vi "Curve fitting.vi"() -> ()   [LabVIEW 2016]
uses:
  <vilib>/Analysis/6fits.llb/Curve Fitting Criteria.ctl
  <vilib>/Analysis/NI_AALPro.lvlib
panel:
  in  "X3":dbl=0.3
  in  "Make it last element ?":bool
  in  "X1":dbl=-0.30000000000000004
  in  "Make it first element ?":bool
  out "Barrier array":dbl[](array[numeric])=[0.3892987340143991]
  in  "X2":dbl
  out "All X for plotting tangent curves":dbl[](array[numeric])=[-0.371549214007658, -8.080417881800293e-06, -0.30000808041805316, 0.29999191958211435, 0.37184895960201303]
  out "XY Graph":cluster{dbl[], dbl[]}[](graph)
  in  "X Array for plotting tangent curves":dbl[](array[numeric])=[0.0, -0.30000000000000004, 0.30000000000000004]
  out "Data section you choose":cluster{dbl[], "Best Polynomial Fit":dbl[]}[](graph)
  in  "Section selection":enum32{"Curve Array section", "Curve section"}(tab)
  in  "Sec of curve array ?":bool=TRUE
  in  "Starting":i32
  in  "length":i32=1
  out "Data array size(s)":i32=6
  in  "length":i32=5012
  in  "Starting":i32=2389
  out "size per curve":i32=4999
  in  "Section of curve ?":bool
  in  "Fitting type":T1(ring)
  in  "method (least square is default)":T2 items=["Least Square", "Least Absolute Residual", "Bisquare"]
  out "Fitting Coefficients":dbl[][](array[numeric])=[[6.3242027435342765e-12, 1.736578525198794e-09, -6.226360766319523e-10, 8.347622973355356e-09, 2.6562376943384554e-08, 1.896167754824949e-07]] format="%#_6p"
  in  "Original data curves":cluster{dbl[], dbl[]}[](graph)=[{array[4999 elements], array[4999 elements]}, {array[4999 elements], array[4999 elements]}, {array[4999 elements], array[4999 elements]}, {array[4999 elements], array[4999 elements]}, {array[4999 elements], array[4999 elements]}, {array[4999 elements], array[4999 elements]}]
  in  "polynomial order":i32=5
  out "Fitting curves":cluster{dbl[], "Best Polynomial Fit":dbl[]}[](graph)
  # "For polynomial fitting: Row is the fitting parameter for each curve (from 0th order to nth order).\nFor exponential fitting: Row is the fitting parameter for each curve (amp, damping, offset -- a,b,c for y=a*exp(bx)+c)."
  # "X difference between intersection of tangent curve at X1 & X2 and intersection of tangent curve at X2 & X3"
  # "Choose range of curve array"
  # "Choose range of each curve"
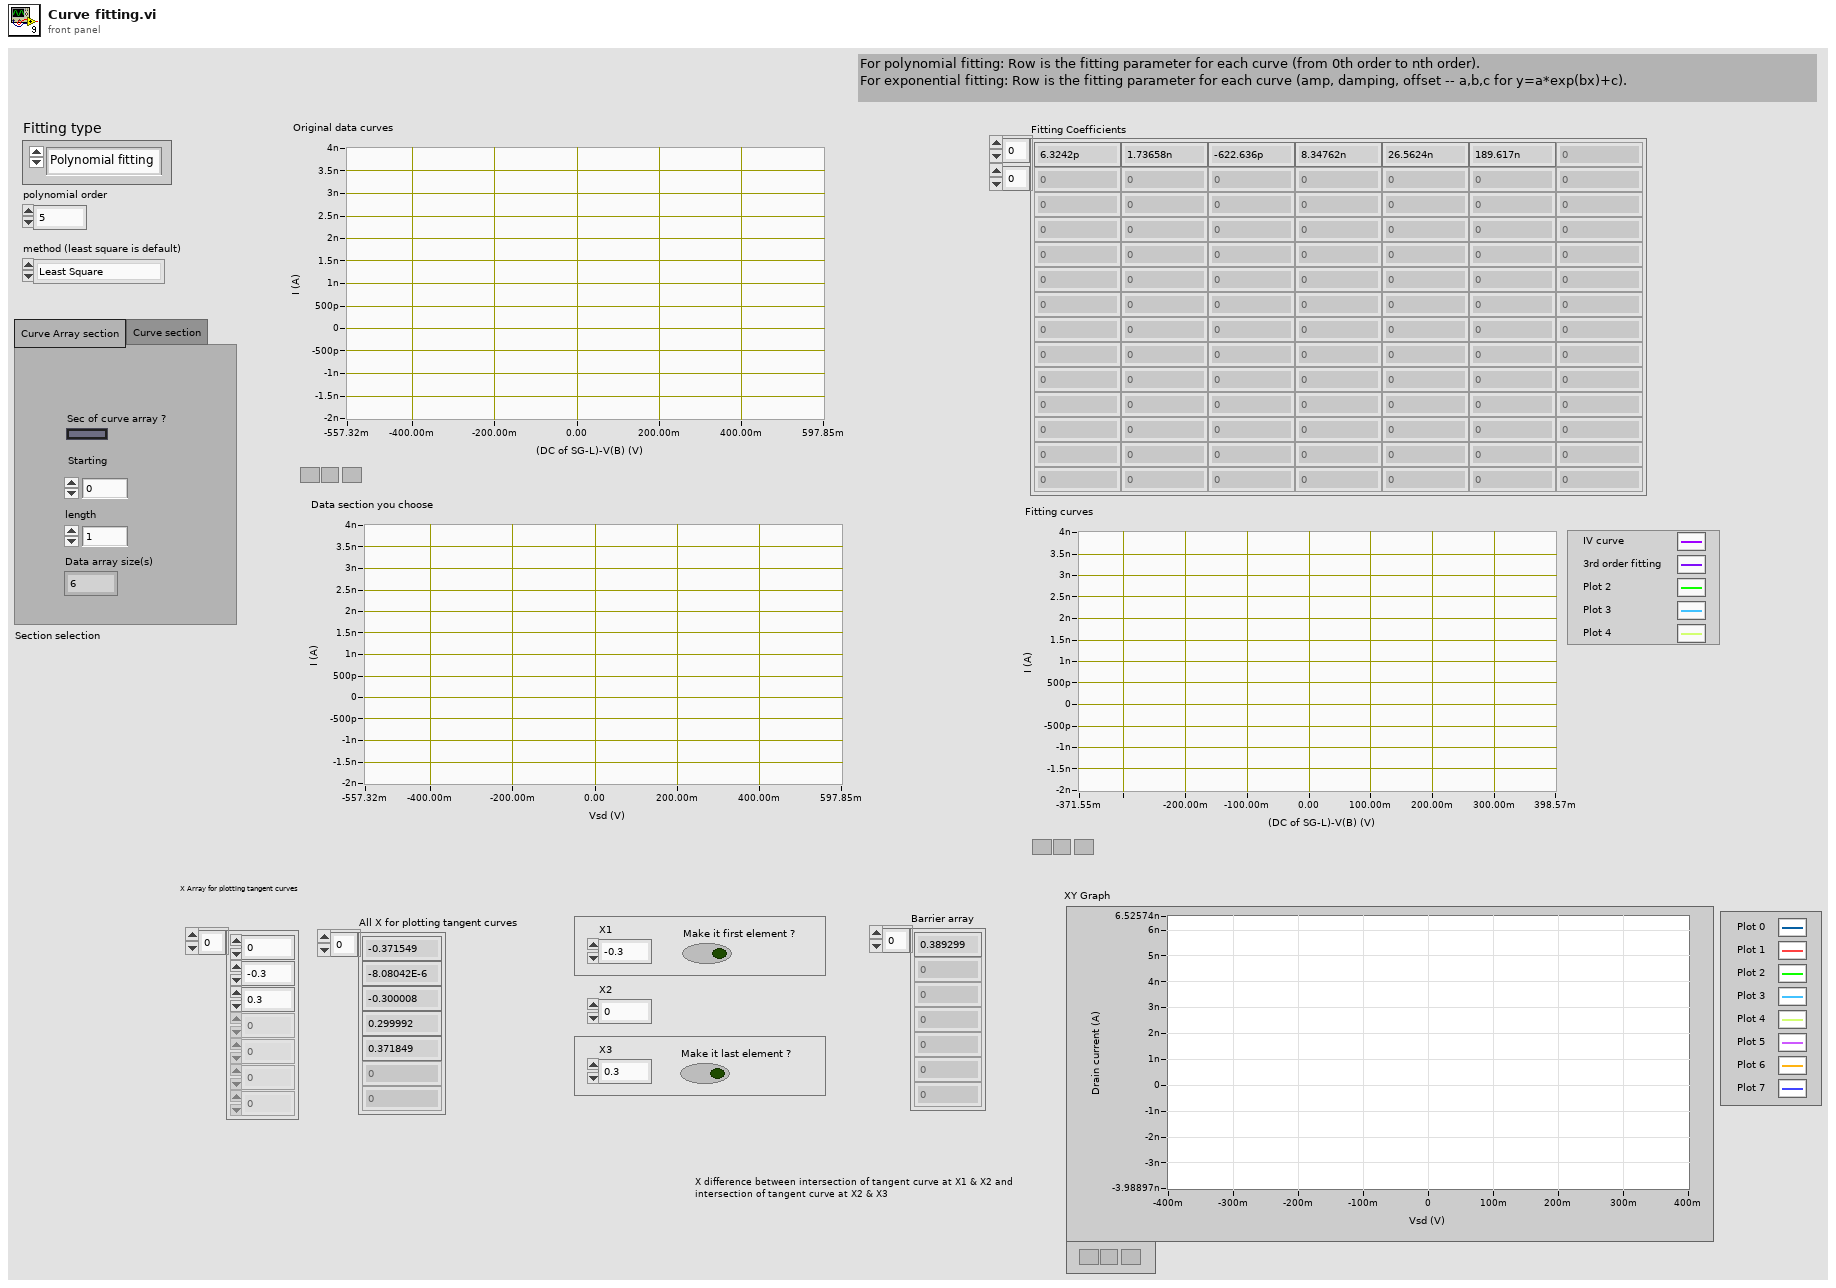
[diagram p1: front panel]
types:
  T1 = enum16{"Polynomial fitting", "Exponential fitting"}
  T2 = typedef "NI_AALPro.lvlib/Curve Fitting Criteria.ctl" = u16
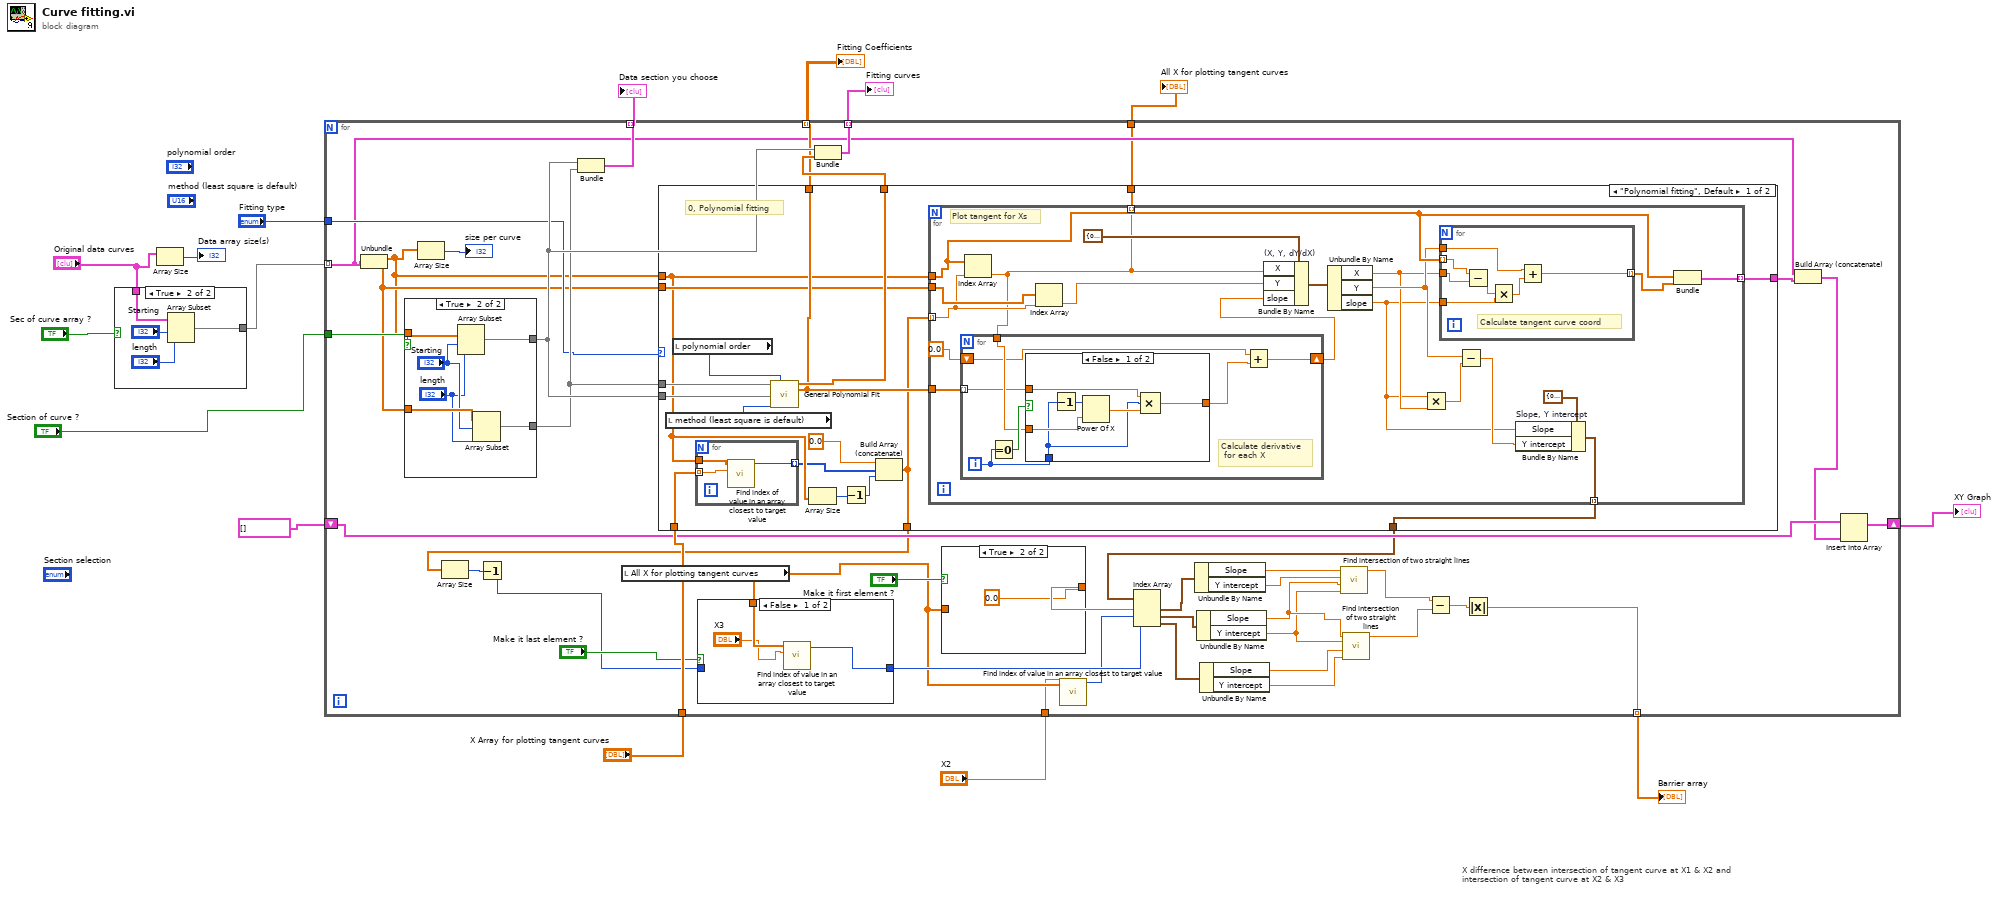
[diagram p0: block diagram]
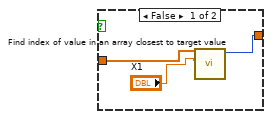
[diagram p4: hidden frame]
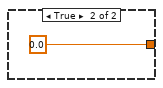
[diagram p5: hidden frame]
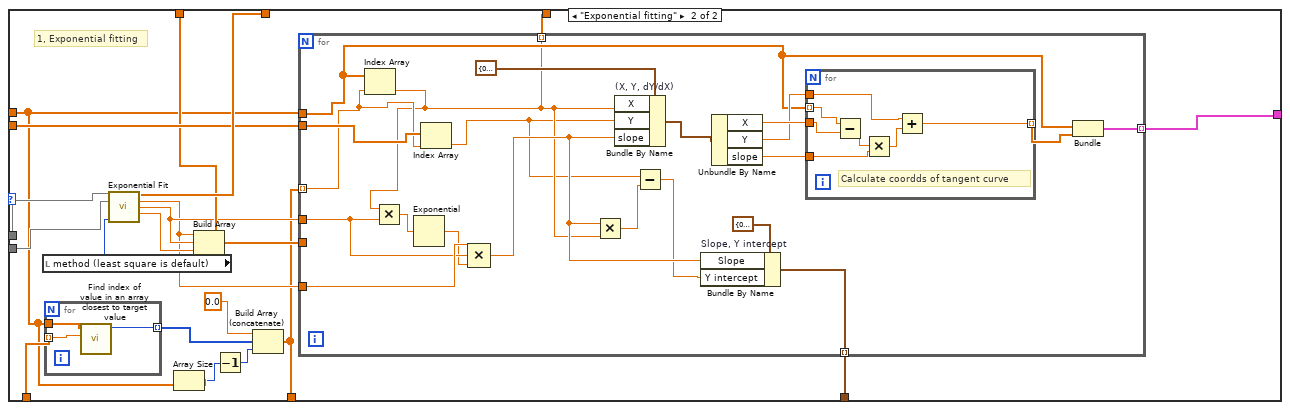
[diagram p6: hidden frame]
diagram:
  # "X difference between intersection of tangent curve at X1 & X2 and intersection of tangent curve at X2 & X3"
  n1 = case shown="True" "Sec of curve array ?" {
    tunnel: "Original data curves" -> [w16 w20]
    tunnel: [w16 w17] -> w10
    frame False {
    }
    frame True {
      n2 = Array Subset(array=w20, index="Starting", length="length") -> (w17:cluster{dbl[], dbl[]}[])
    }
  }
  n3 = Array Size(array="Original data curves") -> (size(s)=→"Data array size(s)":i32)
  n4 = for {
    tunnel: [w54] -> w14 mode=indexing
    tunnel: [w61] -> w15 mode=indexing
    tunnel: w10 -> [w50] mode=indexing
    tunnel: "Fitting type" -> [w53]
    tunnel: "Section of curve ?" -> [w59]
    tunnel: [w56] -> w7 mode=indexing
    tunnel: "X Array for plotting tangent curves" -> [w55]
    shift-right: [w46] -> w4
    shift-left: cluster{dbl[], dbl[]}[] [] ("appended array") -> [w48]
    tunnel: [w45] -> w3
    tunnel: "X2" -> [w23]
    tunnel: [w33] -> w1 mode=indexing
    n5 = Unbundle(w50) -> (w51:dbl[], w52:dbl[])
    n6 = case shown="True" w59 {
      tunnel: w51 -> [w182 w188]
      tunnel: [w182 w187] -> w58
      tunnel: w52 -> [w181 w186]
      tunnel: [w181 w183] -> w57
      frame False {
      }
      frame True {
        n7 = Array Subset(array=w188, index="Starting", length="length") -> (w187:dbl[])
        n8 = Array Subset(array=w186, index="Starting", length="length") -> (w183:dbl[])
      }
    }
    n9 = Array Size(array=w51) -> (size(s)=→"size per curve":i32)
    n10 = Bundle(w58, w57) -> (w56:cluster{dbl[], dbl[]})  [unwired: 1 in]
    n11 = local read "All X for plotting tangent curves"() -> (w25:dbl[])
    n12 = case shown="\"Polynomial fitting\", Default" w53 {
      tunnel: [w87 w145] -> w62
      tunnel: w58 -> [w86 w146]
      tunnel: w57 -> [w85 w147]
      tunnel: w55 -> [w79 w139]
      tunnel: w51 -> [w78 w138]
      tunnel: [w84 w143] -> w54
      tunnel: w52 -> [w81 w144]
      tunnel: [w80 w140] -> w49
      tunnel: [w75 w135] -> w45
      tunnel: [w74 w134] -> w44
      tunnel: [w71 w131] -> w32
      frame "Polynomial fitting", Default {
        # "0, Polynomial fitting"
        n13 = local read "method (least square is default)"() -> (w82:T2)
        n14 = local read "polynomial order"() -> (w83:i32)
        n15 = for {
          tunnel: w79 -> [w90] mode=indexing
          tunnel: w78 -> [w89]
          tunnel: [w88] -> w76 mode=indexing
          n16 = call "Find index of value in an array closest to target value.vi"("Target value"=w90, "Array"=w89) -> ("Index of closest value"=w88:i32)  [unwired: 8 in, 1 out]
        }
        n17 = call <vilib>:"General Polynomial Fit.vi"("Y"=w85, "polynomial order"=w83, "X"=w86, "method"=w82) -> ("Best Polynomial Fit"=w87:dbl[], "Polynomial Coefficients"=w84:dbl[])  [unwired: 8 in, 2 out]
        n18 = Array Size(array=w78) -> (size(s)=w77:i32)
        n19 = Decrement(x=w77) -> (x-1=w73:i32)
        n20 = Build Array (concatenate)(0.0 ("element"), w76, w73) -> (w71:dbl[])
        n21 = for {
          tunnel: w71 -> [w99] mode=indexing
          tunnel: w78 -> [w100]
          tunnel: w81 -> [w109]
          tunnel: w84 -> [w106]
          tunnel: [w101] -> w80 mode=indexing
          tunnel: [w98] -> w75 mode=indexing
          tunnel: [w91] -> w74 mode=indexing
          # "Plot tangent for Xs"
          n22 = Index Array(array=w100, index=w99) -> (element=w98:dbl)
          n23 = for {
            tunnel: w106 -> [w120] mode=indexing
            tunnel: w98 -> [w122]
            shift-right: [w117] -> w104
            shift-left: 0.0 ("Numeric Control") -> [w119]
            i -> [w121]
            # "Calculate derivative\n for each X"
            n24 = Equal To 0?(x=w121) -> (x = 0?=w123:bool)
            n25 = case shown="False" w123 {
              tunnel: w122 -> [w129 _]
              tunnel: w121 -> [w125 _]
              tunnel: w120 -> [w127 _]
              tunnel: [w124 0.0 ("Numeric Control")] -> w118
              frame False {
                n26 = Decrement(x=w125) -> (x-1=w128:i32)
                n27 = Power Of X(1:w129, 2:w128) -> (0:w126:dbl)
                n28 = Compound Arithmetic op=MULTIPLY(w127, w125, w126) -> (w124:dbl)
              }
              frame True {
              }
            }
            n29 = Add(x=w119, y=w118) -> (x+y=w117:dbl)
          }
          n30 = Index Array(array=w109, index=w99) -> (element=w107:dbl)
          n31 = Bundle By Name "(X, Y, dY/dX)"(cluster=cluster{"X":dbl, "Y":dbl, "slope":dbl} {"X"=0.0, "Y"=0.0, "slope"=0.0}, "X"=w98, "Y"=w107, "slope"=w104) -> (w103:cluster{"X":dbl, "Y":dbl, "slope":dbl})
          n32 = Unbundle By Name(w103) -> ("X"=w93:dbl, "Y"=w94:dbl, "slope"=w92:dbl)
          n33 = Multiply(x=w92, y=w93) -> (x*y=w96:dbl)
          n34 = for {
            tunnel: w100 -> [w116] mode=indexing
            tunnel: w93 -> [w115]
            tunnel: w92 -> [w114]
            tunnel: w94 -> [w112]
            tunnel: [w110] -> w102 mode=indexing
            # "Calculate tangent curve coord"
            n35 = Subtract(x=w116, y=w115) -> (x-y=w113:dbl)
            n36 = Multiply(x=w113, y=w114) -> (x*y=w111:dbl)
            n37 = Add(x=w112, y=w111) -> (x+y=w110:dbl)
          }
          n38 = Subtract(x=w94, y=w96) -> (x-y=w95:dbl)
          n39 = Bundle By Name "Slope, Y intercept"(cluster=cluster{"Slope":dbl, "Y intercept":dbl} {"Slope"=0.0, "Y intercept"=0.0}, "Slope"=w92, "Y intercept"=w95) -> (w91:cluster{"Slope":dbl, "Y intercept":dbl})
          n40 = Bundle(w100, w102) -> (w101:cluster{dbl[], dbl[]})  [unwired: 1 in]
        }
      }
      frame "Exponential fitting" {
        # "1, Exponential fitting"
        n41 = local read "method (least square is default)"() -> (w148:T2)
        n42 = for {
          tunnel: w139 -> [w152] mode=indexing
          tunnel: w138 -> [w151]
          tunnel: [w150] -> w137 mode=indexing
          n43 = call "Find index of value in an array closest to target value.vi"("Target value"=w152, "Array"=w151) -> ("Index of closest value"=w150:i32)  [unwired: 8 in, 1 out]
        }
        n44 = call <vilib>:"Exponential Fit.vi"("Y"=w147, "X"=w146, "method"=w148) -> ("Best Exponential Fit"=w145:dbl[], "amplitude"=w141:dbl, "damping"=w142:dbl, "offset"=w149:dbl)  [unwired: 7 in, 2 out]
        n45 = Array Size(array=w138) -> (size(s)=w136:i32)
        n46 = Build Array(w141, w142, w149) -> (w143:dbl[])
        n47 = Decrement(x=w136) -> (x-1=w133:i32)
        n48 = Build Array (concatenate)(0.0 ("element"), w137, w133) -> (w131:dbl[])
        n49 = for {
          tunnel: w131 -> [w160] mode=indexing
          tunnel: w138 -> [w161]
          tunnel: w144 -> [w173]
          tunnel: w143 -> [_]
          tunnel: w142 -> [w169]
          tunnel: w141 -> [w170]
          tunnel: [w162] -> w140 mode=indexing
          tunnel: [w157] -> w135 mode=indexing
          tunnel: [w153] -> w134 mode=indexing
          n50 = Index Array(array=w161, index=w160) -> (element=w157:dbl)
          n51 = Multiply(x=w157, y=w169) -> (x*y=w171:dbl)
          n52 = Exponential(1:w171) -> (0:w168:dbl)
          n53 = Index Array(array=w173, index=w160) -> (element=w155:dbl)
          n54 = Compound Arithmetic op=MULTIPLY(w170, w169, w168) -> (w158:dbl)
          n55 = Multiply(x=w158, y=w157) -> (x*y=w156:dbl)
          n56 = Bundle By Name "(X, Y, dY/dX)"(cluster=cluster{"X":dbl, "Y":dbl, "slope":dbl} {"X"=0.0, "Y"=0.0, "slope"=0.0}, "X"=w157, "Y"=w155, "slope"=w158) -> (w163:cluster{"X":dbl, "Y":dbl, "slope":dbl})
          n57 = Subtract(x=w155, y=w156) -> (x-y=w154:dbl)
          n58 = Bundle By Name "Slope, Y intercept"(cluster=cluster{"Slope":dbl, "Y intercept":dbl} {"Slope"=0.0, "Y intercept"=0.0}, "Slope"=w158, "Y intercept"=w154) -> (w153:cluster{"Slope":dbl, "Y intercept":dbl})
          n59 = Unbundle By Name(w163) -> ("X"=w167:dbl, "Y"=w165:dbl, "slope"=w166:dbl)
          n60 = for {
            tunnel: w161 -> [w180] mode=indexing
            tunnel: w167 -> [w179]
            tunnel: w166 -> [w178]
            tunnel: w165 -> [w176]
            tunnel: [w174] -> w164 mode=indexing
            # "Calculate coordds of tangent curve"
            n61 = Subtract(x=w180, y=w179) -> (x-y=w177:dbl)
            n62 = Multiply(x=w177, y=w178) -> (x*y=w175:dbl)
            n63 = Add(x=w176, y=w175) -> (x+y=w174:dbl)
          }
          n64 = Bundle(w161, w164) -> (w162:cluster{dbl[], dbl[]})  [unwired: 1 in]
        }
      }
    }
    n65 = Array Size(array=w32) -> (size(s)=w31:i32)
    n66 = Decrement(x=w31) -> (x-1=w26:i32)
    n67 = case shown="False" "Make it last element ?" {
      tunnel: w26 -> [_ w66]
      tunnel: [w63 w66] -> w28
      tunnel: w25 -> [w65 _]
      frame False {
        n68 = call "Find index of value in an array closest to target value.vi"("Target value"="X3", "Array"=w65) -> ("Index of closest value"=w63:i32)  [unwired: 8 in, 1 out]
      }
      frame True {
      }
    }
    n69 = Bundle(w58, "Best Exponential Fit"=w62) -> (w61:cluster{dbl[], "Best Exponential Fit":dbl[]})  [unwired: 1 in]
    n70 = case shown="True" "Make it first element ?" {
      tunnel: [w67 0.0 ("element")] -> w29
      tunnel: w25 -> [w69 _]
      frame False {
        n71 = call "Find index of value in an array closest to target value.vi"("Target value"="X1", "Array"=w69) -> ("Index of closest value"=w67:i32)  [unwired: 8 in, 1 out]
      }
      frame True {
      }
    }
    n72 = call "Find index of value in an array closest to target value.vi"("Target value"=w23, "Array"=w25) -> ("Index of closest value"=w24:i32)  [unwired: 8 in, 1 out]
    n73 = Index Array(array=w44, index #1=w29, index #2=w24, index #3=w28) -> (element #1=w43:cluster{"Slope":dbl, "Y intercept":dbl}, element #2=w42:cluster{"Slope":dbl, "Y intercept":dbl}, element #3=w41:cluster{"Slope":dbl, "Y intercept":dbl})
    n74 = Unbundle By Name(w43) -> ("Slope"=w40:dbl, "Y intercept"=w39:dbl)
    n75 = Unbundle By Name(w42) -> ("Slope"=w22:dbl, "Y intercept"=w21:dbl)
    n76 = Unbundle By Name(w41) -> ("Slope"=w38:dbl, "Y intercept"=w37:dbl)
    n77 = call "Find intersection of two straight lines.vi"("Intercept 1"=w21, "Slope 1"=w22, "Intercept 0"=w39, "Slope 0"=w40) -> ("X of intersection"=w36:dbl)  [unwired: 6 in, 1 out]
    n78 = call "Find intersection of two straight lines.vi"("Intercept 1"=w37, "Slope 1"=w38, "Intercept 0"=w21, "Slope 0"=w22) -> ("X of intersection"=w35:dbl)  [unwired: 6 in, 1 out]
    n79 = Subtract(x=w36, y=w35) -> (x-y=w34:dbl)
    n80 = Absolute Value(x=w34) -> (abs(x)=w33:dbl)
    n81 = Build Array (concatenate)(w50, w49) -> (w47:cluster{dbl[], dbl[]}[])
    n82 = Insert Into Array(array=w48, new element=w47) -> (w46:cluster{dbl[], dbl[]}[])  [unwired: 1 in]
  }
  "Fitting curves" <- w15
  "Fitting Coefficients" <- w14
  "Data section you choose" <- w7
  "XY Graph" <- w4
  "All X for plotting tangent curves" <- w3
  "Barrier array" <- w1
